vi "32 Audio and FFT's.vi"() -> ()   [LabVIEW 2019]
uses:
  _Subs/OpenDiagram/Open_XControl.xctl
  <vilib>/Analysis/2dsp.llb/Real FFT.vi
  <vilib>/measure/maspectr.llb/FFT Power Spectrum and PSD for 1 Chan.vi
  <vilib>/express/express analysis/Spectral/Block/exnSpectralBlock spectral measurements power poly.vi
  <vilib>/express/express analysis/Spectral/Block/exnSpectralBlock spectral measurements power DDT.vi
  <vilib>/express/express analysis/Spectral/XNode/ExpressSpectralMeasurementsBlockNode.xnode
  <vilib>/Analysis/NI_AALPro.lvlib
  <vilib>/measure/NI_MAPro.lvlib
panel:
  in  "Tab Control":T1(tab)
  in  "Duration (s)":dbl=1.0
  in  "Sample rate (Hz)":dbl=44100.0
  out "Sound Wave of Audio Snippet":dynamicdata(graph) caption="Data"
  in  "FFT size":i32=-1
  out "Spectral Measurements FFT Graph":dynamicdata(graph)
  in  "Path":path
  out ".wav file sound wave Graph":waveform(dbl)(graph)
  out "FFT of .wav file Graph":cluster{"f0":dbl, "df":dbl, "magnitude":dbl[]}(graph)
  out "FFT Function Graph":dbl[](graph)
  in  "OpenDiag":refnum<vi>(xcontrol)
  # "32 Audio and FFT's\nThis code uses the acquire sound and read .wav file functions, and also provides a few \ndifferent ways to create Fourier Transforms.  \n\nInstructions:\n1. Select a .wav file from your computer by hitting the folder icon next to Path. \n2. Hit run to plot the sound wave on the first graph. The second graph shows the FFT of that file. \n3. Hit run again to record a snippet of audio and see how the waveform is displayed (graph #3). Immediately \nbelow are two FFTs of that audio snippet. \n4. Play around with the duration length, sample rate, and FFT size. How do things change? \n5. Look at the block diagram and compare how the FFT data is created for each graph."
  # "For more details on the math behind Fourier Transforms, watch this video!\nhttps://www.youtube.com/watch?v=spUNpyF58BY"
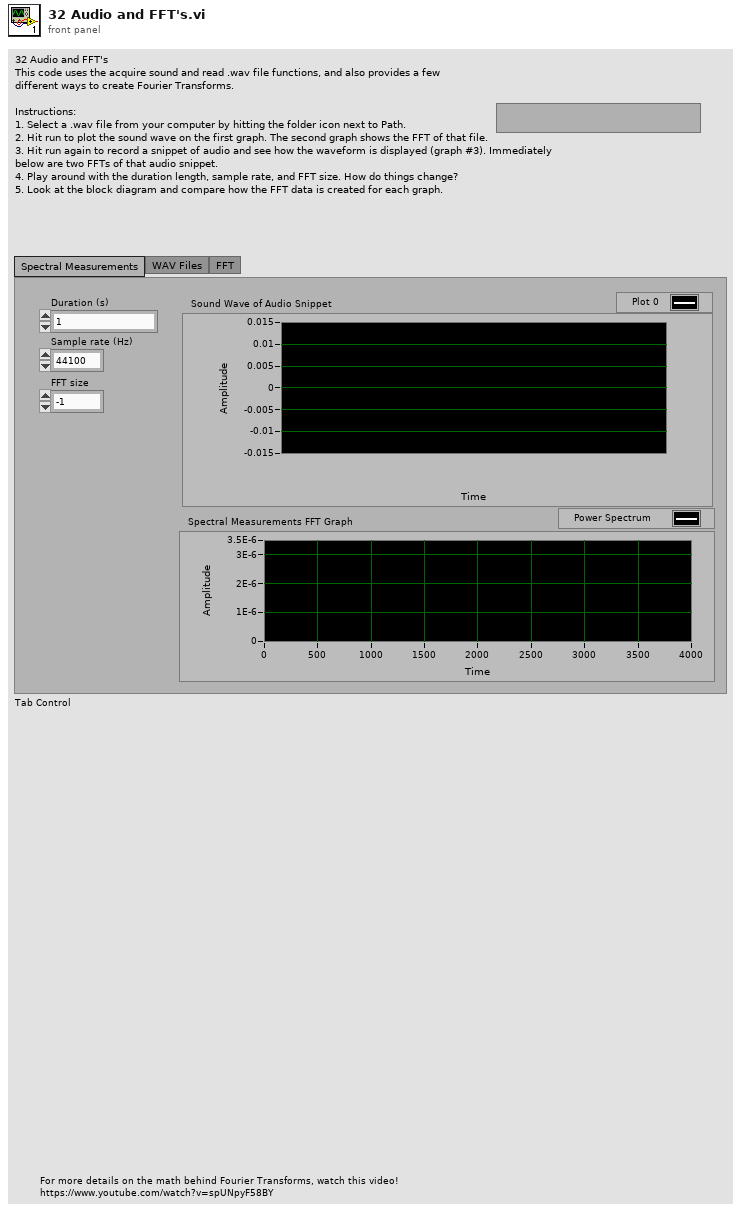
[diagram p1: front panel]
types:
  T1 = enum32{"Spectral Measurements", "WAV Files", "FFT"}
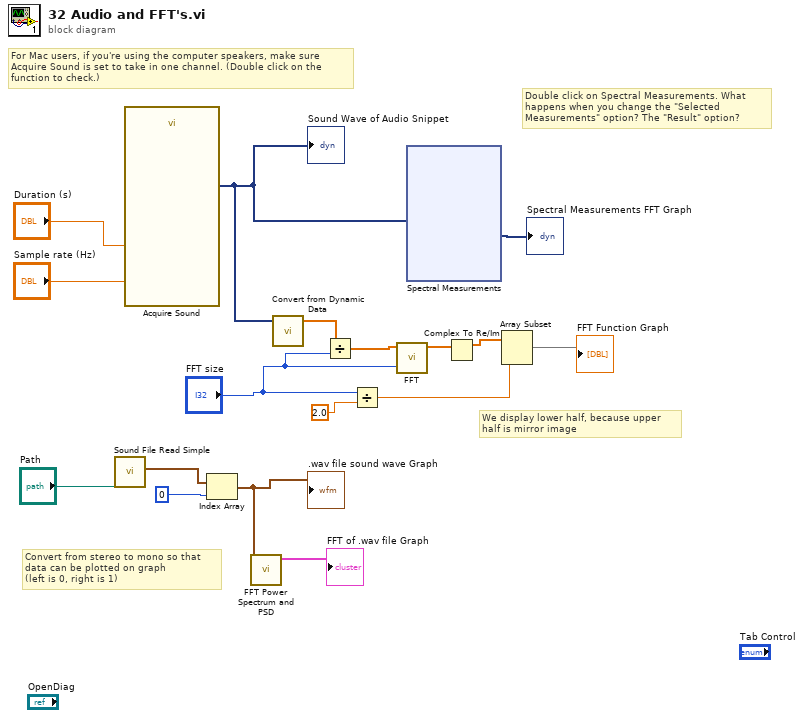
[diagram p0: block diagram]
diagram:
  # "Double click on Spectral Measurements. What \nhappens when you change the \"Selected \nMeasurements\" option? The \"Result\" option?"
  # "Convert from stereo to mono so that \ndata can be plotted on graph\n(left is 0, right is 1)"
  # "We display lower half, because upper \nhalf is mirror image"
  # "For Mac users, if you're using the computer speakers, make sure\nAcquire Sound is set to take in one channel. (Double click on the \nfunction to check.)"
  n1 = call <vilib>:"Sound File Read Simple.vi"("path"="Path") -> ("data"=w4:waveform(dbl)[])  [unwired: 7 in, 3 out]
  n2 = call "Acquire Sound"("Duration (s)"="Duration (s)", "Sample rate (Hz)"="Sample rate (Hz)") -> ("Data"=w12:dynamicdata)  [unwired: 16 in, 1 out]
  "Sound Wave of Audio Snippet" <- w12
  n3 = Index Array(array=w4, index=0) -> (element=w1:waveform(dbl))
  ".wav file sound wave Graph" <- w1
  n4 = call-poly <vilib>:"FFT Power Spectrum and PSD.vi"("time signal"=w1) -> ("Power Spectrum / PSD"=→"FFT of .wav file Graph":cluster{"f0":dbl, "df":dbl, "magnitude":dbl[]})  [unwired: 7 in, 3 out]
  n5 = call "Convert from Dynamic Data"("Dynamic Data Type"=w12) -> ("Array"=w11:dbl[])  [unwired: 3 in]
  n6 = Divide(x=w11, y="FFT size") -> (x/y=w10:dbl[])
  n7 = Divide(x="FFT size", y=2.0) -> (x/y=w6:dbl)
  n8 = call-poly <vilib>:"FFT.vi"("FFT size"="FFT size", "X"=w10) -> ("FFT {X}"=w9:cdb[])  [unwired: 8 in, 1 out]
  n9 = xnode "Spectral Measurements"("Signals"=w12) -> ("Power Spectrum"=→"Spectral Measurements FFT Graph":dynamicdata)  [unwired: 1 in, 1 out]
  n10 = Complex To Re/Im(x + iy=w9) -> (x=w14:dbl[])  [unwired: 1 out]
  n11 = Array Subset(array=w14, length=w6) -> (→"FFT Function Graph":dbl[])  [unwired: 1 in]
